vi "Path-Find_Start_Finish.vi"(11 "Tile Array":T2[][](array[typedef])) -> (2 "Start":T1, 3 "Finish":T1)   [LabVIEW 2020]
doc: "<B>Description:</B> Scans the Tile Array for the start and the finish Tiles.\n\n<B>Date:</B> 06/2019\n<B>Author:</B> Luke Jarocki, Choose Movement Consulting, LLC"
uses:
  Controls/TileColor.ctl
  Controls/Parse-(X,Y).ctl
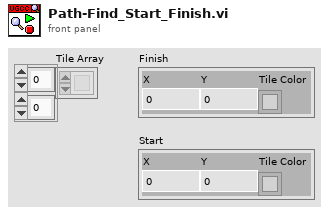
[diagram p1: front panel]
types:
  T1 = typedef "Parse-(X,Y).ctl" = cluster{"X":i32, "Y":i32, "Tile Color":T2}
  T2 = typedef "TileColor.ctl" = u16
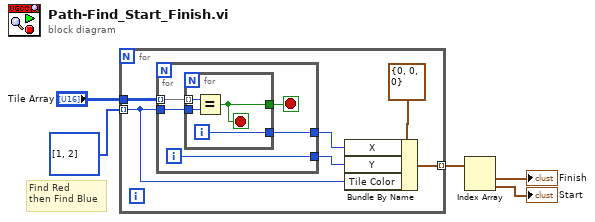
[diagram p0: block diagram]
diagram:
  # "Find Red\nthen Find Blue"
  n1 = for {
    tunnel: "Tile Array" -> [w11]
    tunnel: T2[] [1, 2] -> [w9] mode=indexing
    tunnel: [w6] -> w2 mode=indexing
    n2 = for {
      tunnel: w11 -> [w16] mode=indexing
      tunnel: [w15] -> w8
      tunnel: [w14] -> w7
      tunnel: w9 -> [w12]
      i -> [w14]
      stop <- w13 stop-if-true
      n3 = for {
        tunnel: w16 -> [w20] mode=indexing
        tunnel: [w19] -> w15
        tunnel: [w18] -> w13
        tunnel: w12 -> [w17]
        i -> [w19]
        stop <- w18 stop-if-true
        n4 = Equal?(x=w20, y=w17) -> (x = y?=w18:bool)
      }
    }
    n5 = Bundle By Name(cluster=T1 {"X"=0, "Y"=0, "Tile Color"=0} ("(X,Y)"), "X"=w8, "Y"=w7, "Tile Color"=w9) -> (w6:T1)
  }
  n6 = Index Array(array=w2) -> (element #1=→"Finish":T1, element #2=→"Start":T1)  [unwired: 2 in]
